vi "libssh2_channel_open_ex.vi"(5 "packet_size (32 KiB)":u32=32768, 7 "window_size (2 MiB)":u32=2097152, 8 "error in (no error)":errorcluster, 9 "message":string, 10 "channel_type":string="session", 11 "session":T1) -> (0 "error out":errorcluster, 3 "channel":T2)   [LabVIEW 2013, in "libssh2.lvlib"]
doc: "Establishes a new channel."
uses:
  libssh2.lvlib
  Channel Refnum.ctl
  Session Refnum.ctl
  libssh2.dll
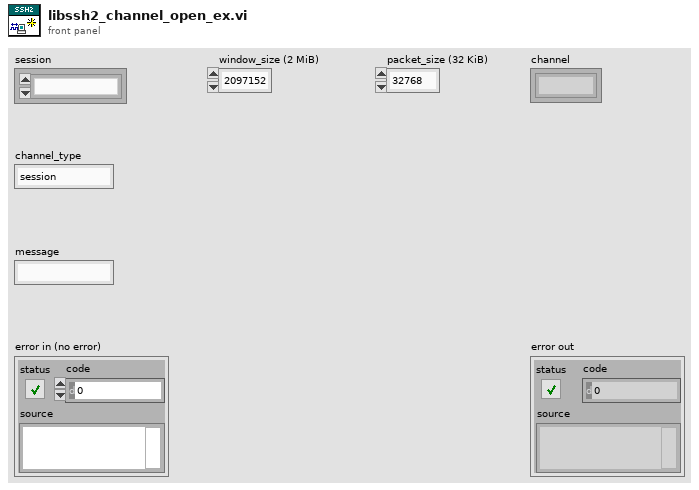
[diagram p1: front panel]
types:
  T1 = typedef "libssh2.lvlib/Session Refnum.ctl" = refnum<k1>
  T2 = typedef "libssh2.lvlib/Channel Refnum.ctl" = refnum<k1>
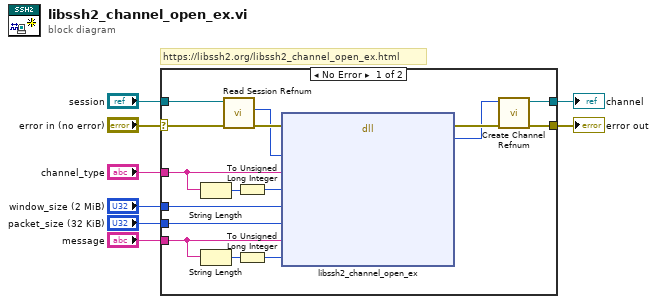
[diagram p0: block diagram]
diagram:
  # "https://libssh2.org/libssh2_channel_open_ex.html"
  n1 = case shown="No Error" "error in (no error)" {
    selector: "error in (no error)" -> [w9 w25]
    tunnel: "window_size (2 MiB)" -> [w23 _]
    tunnel: "packet_size (32 KiB)" -> [w22 _]
    tunnel: "message" -> [w20 _]
    tunnel: "channel_type" -> [w18 _]
    tunnel: "session" -> [w14 _]
    tunnel: [w12 w25] -> w3
    tunnel: [w10 _] -> w2
    frame No Error {
      n2 = String Length(string=w18) -> (length=w16:i32)
      n3 = String Length(string=w20) -> (length=w17:i32)
      n4 = call "Read Session Refnum.vi"("error in (no error)"=w9, "session"=w14) -> ("error out"=w15:errorcluster, "LIBSSH2_SESSION*"=w13:u64)  [unwired: 8 in]
      n5 = To Unsigned Long Integer(number=w16) -> (unsigned 32bit integer=w24:u32)
      n6 = To Unsigned Long Integer(number=w17) -> (unsigned 32bit integer=w19:u32)
      n7 = dll-call lib="C:/Users/pasca/source/repos/libssh2-labview/libssh2/libssh2**.*" fn="libssh2_channel_open_ex"(error in=w15, "session"=w13, "channel_type"=w18, "channel_type_len"=w24, "window_size"=w23, "packet_size"=w22, "message"=w20, "message_len"=w19) -> (error out=w21:errorcluster, "return value"=w11:u64)  [unwired: 9 in, 1 out]
      n8 = call "Create Channel Refnum.vi"("error in (no error)"=w21, "LIBSSH2_CHANNEL*"=w11) -> ("error out"=w12:errorcluster, "channel"=w10:T2)  [unwired: 8 in]
    }
    frame Error {
    }
  }
  "channel" <- w2
  "error out" <- w3
